vi "Dia 1 - clusters.vi"() -> ()   [LabVIEW 2014]
panel:
  out "output variable 2":dbl
  out "output variable":dbl
  out "Num":i32
  out "Array":i32[](array[numeric])
  out "Boolean":bool
  out "Cluster":T1 {"Knob" scale=0.0..10.0}
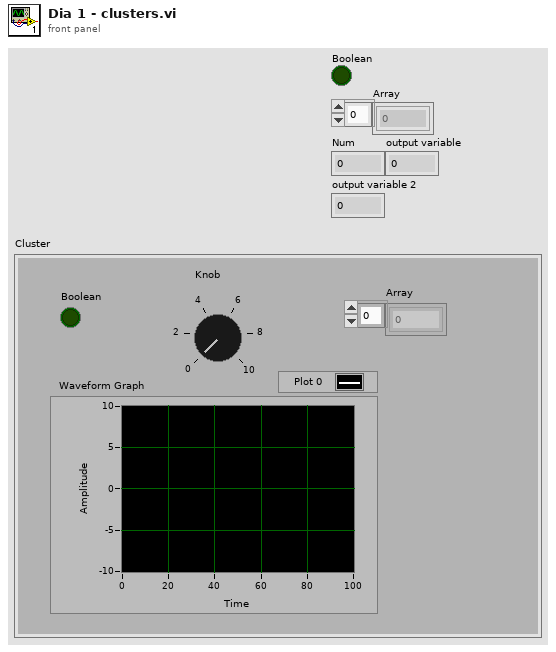
[diagram p1: front panel]
types:
  T1 = cluster{"Array":dbl[], "Boolean":bool, "Waveform Graph":dbl[], "Knob":dbl}
  T2 = cluster{"Array":i32[], "Num":i32, "Boolean":bool, "Double":dbl}
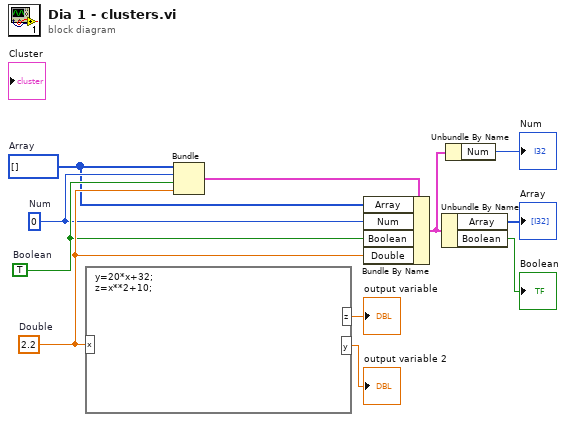
[diagram p0: block diagram]
diagram:
  w4 = 2.2  # Double
  w1 = i32[] []  # Array
  w3 = TRUE  # Boolean
  w2 = 0  # Num
  n1 = formula code="y=20*x+32;\nz=x**2+10;"("x"=w4) -> ("y"=→"output variable 2":dbl, "z"=→"output variable":dbl)
  n2 = Bundle("Array"=w1, "Num"=w2, "Boolean"=w3, "Double"=w4) -> (w11:T2)  [unwired: 1 in]
  n3 = Bundle By Name(cluster=w11, "Array"=w1, "Num"=w2, "Boolean"=w3, "Double"=w4) -> (w8:T2)
  n4 = Unbundle By Name(w8) -> ("Array"=→"Array":i32[], "Boolean"=→"Boolean":bool)
  n5 = Unbundle By Name(w8) -> ("Num"=→"Num":i32)
